vi "runCM.vi"() -> ()   [LabVIEW 2009, in "run.lvlib"]
uses:
  run.lvlib
  IntegrationManagement/CameraManager.lvclass
  Tools/Filing/FileSystem/FileSystem.lvclass
  Tools/Filing/FileNeologist/FileNeologist.lvclass
  Tools/Filing.lvlib
panel:
  in  "Hardware Connected?":bool
  out "ready":bool
  in  "Camera":enum16{"AndorIKon", "ICCamera"}(ring)
  in  "stop":bool
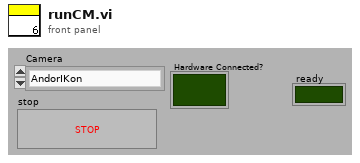
[diagram p1: front panel]
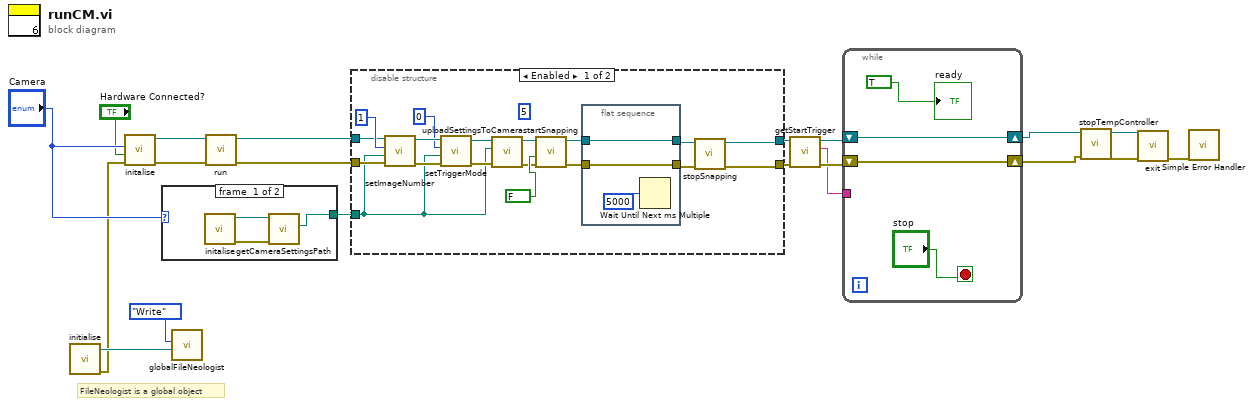
[diagram p0: block diagram]
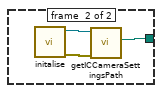
[diagram p3: hidden frame]
diagram:
  # "FileNeologist is a global object"
  n1 = call "initialise.vi"() -> ("error out"=w6:errorcluster, "FileNeologist out"=w8:refnum<class "FileNeologist.lvclass">)  [unwired: 10 in]
  n2 = call "initalise.vi"("error in (no error)"=w6, "Hardware Connected?"="Hardware Connected?", "Camera"="Camera") -> ("error out"=w19:errorcluster, "CameraManager out"=w20:refnum<class "CameraManager.lvclass">)  [unwired: 7 in]
  n3 = case shown="\"AndorIKon\", Default" "Camera" {
    tunnel: [w21 w26] -> w15
    frame #0 {
      n4 = call "initalise.vi"() -> ("error out"=w23:errorcluster, "FileSystem out"=w22:refnum<class "FileSystem.lvclass">)  [unwired: 10 in]
      n5 = call-dynamic "getCameraSettingsPath.vi"("error in (no error)"=w23, "FileSystem.lvclass in"=w22) -> ("CameraSettingsPath"=w21:path)  [unwired: 7 in, 2 out]
    }
    frame #1 {
      n6 = call "initalise.vi"() -> ("error out"=w25:errorcluster, "FileSystem out"=w24:refnum<class "FileSystem.lvclass">)  [unwired: 10 in]
      n7 = call-dynamic "getICCameraSettingsPath.vi"("error in (no error)"=w25, "FileSystem.lvclass in"=w24) -> ("ICCameraSettingsPath"=w26:path)  [unwired: 7 in, 2 out]
    }
  }
  n8 = call "globalFileNeologist.vi"("FileNeologist in"=w8, "Action"=enum16{"Write", "Read"}."Write") -> ()  [unwired: 9 in, 1 out]
  n9 = call-dynamic "run.vi"("error in (no error)"=w19, "CameraManager in"=w20) -> ("error out"=w16:errorcluster, "CameraManager out"=w17:refnum<class "CameraManager.lvclass">)  [unwired: 8 in]
  n10 = disable-structure shown="Enabled" {
    disable-tunnel: w17 -> [w43 w49]
    disable-tunnel: w16 -> [w42 w48]
    disable-tunnel: w15 -> [w36 _]
    disable-tunnel: [w28 w49] -> w12
    disable-tunnel: [w27 w48] -> w13
    frame #0 {
      (unwired) 5
      n11 = call "setImageNumber.vi"("error in (no error)"=w42, "Path"=w36, "imageNumber"=1, "CameraManager in"=w43) -> ("error out"=w40:errorcluster, "CameraManager out"=w41:refnum<class "CameraManager.lvclass">)  [unwired: 6 in]
      n12 = call "setTriggerMode.vi"("error in (no error)"=w40, "Path"=w36, "triggerMode"=0, "CameraManager in"=w41) -> ("error out"=w37:errorcluster, "CameraManager out"=w38:refnum<class "CameraManager.lvclass">)  [unwired: 6 in]
      n13 = call "uploadSettingsToCamera.vi"("error in (no error)"=w37, "Path"=w36, "CameraManager in"=w38) -> ("error out"=w33:errorcluster, "CameraManager out"=w34:refnum<class "CameraManager.lvclass">)  [unwired: 7 in]
      n14 = call "startSnapping.vi"("error in (no error)"=w33, "releaseWhenReady"=FALSE, "CameraManager in"=w34) -> ("error out"=w31:errorcluster, "CameraManager out"=w32:refnum<class "CameraManager.lvclass">)  [unwired: 7 in]
      n15 = flat-sequence {
        tunnel: w32 -> [w45]
        tunnel: w31 -> [w46]
        tunnel: [w46] -> w29
        tunnel: [w45] -> w30
        frame #0 {
          n16 = Wait Until Next ms Multiple(millisecond multiple=5000) -> ()  [unwired: 1 out]
        }
      }
      n17 = call-dynamic "stopSnapping.vi"("error in (no error)"=w29, "CameraManager in"=w30) -> ("error out"=w27:errorcluster, "CameraManager out"=w28:refnum<class "CameraManager.lvclass">)  [unwired: 8 in]
    }
    frame #1 {
    }
  }
  n18 = call-dynamic "getStartTrigger.vi"("error in (no error)"=w13, "CameraManager in"=w12) -> ("error out"=w14:errorcluster, "start_trigger"=w10:string, "CameraManager out"=w11:refnum<class "CameraManager.lvclass">)  [unwired: 7 in]
  n19 = while {
    shift-right: [w53] -> w4
    shift-left: w11 -> [w53]
    shift-right: [w52] -> w3
    shift-left: w14 -> [w52]
    tunnel: w10 -> [_]
    stop <- "stop" stop-if-true
    "ready" <- TRUE
  }
  n20 = call "stopTempController.vi"("error in (no error)"=w3, "CameraManager in"=w4) -> ("error out"=w1:errorcluster, "CameraManager out"=w2:refnum<class "CameraManager.lvclass">)  [unwired: 8 in]
  n21 = call-dynamic "exit.vi"("error in (no error)"=w1, "CameraManager in"=w2) -> ("error out"=w9:errorcluster)  [unwired: 8 in, 1 out]
  n22 = call <vilib>:"Simple Error Handler.vi"("error in (no error)"=w9) -> ()  [unwired: 4 in, 5 out]
